vi "set Clock Free Running.vi"(10 "Free Running":bool, 11 "Clock Generator in":refnum<class "IO.lvclass">) -> (3 "Clock Generator out":refnum<class "IO.lvclass">)   [LabVIEW 2021, in "IO.lvclass"]
uses:
  IO.lvclass
  IO.lvclass/IO.ctl
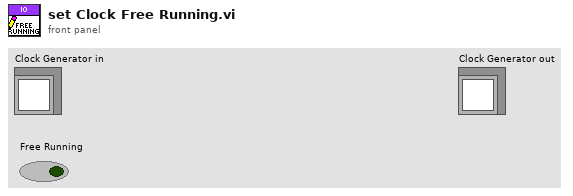
[diagram p1: front panel]
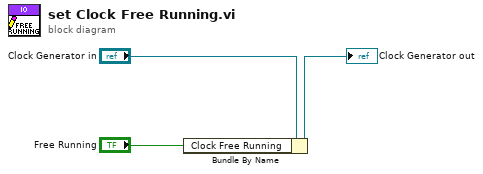
[diagram p0: block diagram]
diagram:
  n1 = Bundle By Name(cluster="Clock Generator in", "Clock Free Running"="Free Running") -> (→"Clock Generator out":refnum<class "IO.lvclass">)
